vi "Quaternion_Equals.vi"(9 "Other Quaternion":T1={"R"=1.0, "V"=[0.0, 0.0, 0.0]}, 11 "Quaternion":T1={"R"=1.0, "V"=[0.0, 0.0, 0.0]}) -> (1 "Equal2":bool, 3 "Equal":bool)   [LabVIEW 2019, in "Trajectory_Library.lvlib"]
doc: "Convenience constructors that takes in x and y values directly instead of having to construct a Translation2d.\n\nParameters:\n - X- The x component of the translational component of the pose.\n - Y - The y component of the translational component of the pose.\n - Rotation (Heading) - The rotational component of the pose.\n\nReturns:\n - OUT POSE - Output POSE"
uses:
  Trajectory_Library.lvlib
  QUATERNION.ctl
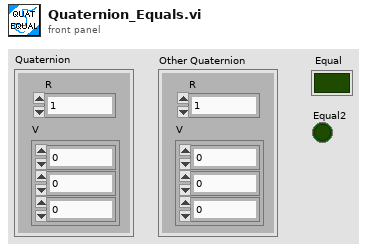
[diagram p1: front panel]
types:
  T1 = typedef "Trajectory_Library.lvlib/QUATERNION.ctl" = cluster{"R":dbl, "V":dbl[]}
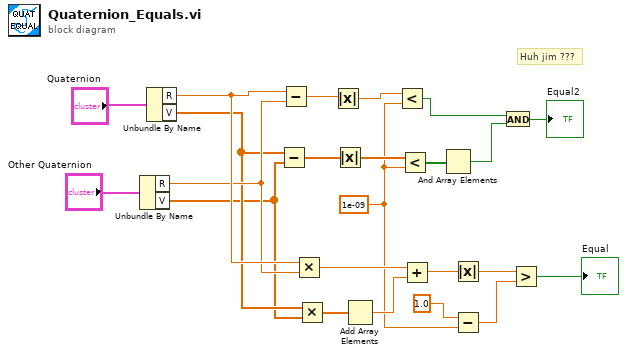
[diagram p0: block diagram]
diagram:
  w4 = 1e-09 ("y")
  # "Huh jim ???"
  n1 = Unbundle By Name("Other Quaternion") -> ("R"=w13:dbl, "V"=w11:dbl[])
  n2 = Unbundle By Name("Quaternion") -> ("R"=w14:dbl, "V"=w12:dbl[])
  n3 = Subtract(x=w12, y=w11) -> (x-y=w20:dbl[])
  n4 = Subtract(x=w14, y=w13) -> (x-y=w21:dbl)
  n5 = Multiply(x=w14, y=w13) -> (x*y=w9:dbl)
  n6 = Multiply(x=w12, y=w11) -> (x*y=w10:dbl[])
  n7 = Absolute Value(x=w21) -> (abs(x)=w19:dbl)
  n8 = Absolute Value(x=w20) -> (abs(x)=w18:dbl[])
  n9 = Add Array Elements(numeric array=w10) -> (sum=w8:dbl)
  n10 = Less?(x=w19, y=w4) -> (x < y?=w17:bool)
  n11 = Less?(x=w18, y=w4) -> (x < y?=w16:bool[])
  n12 = Add(x=w9, y=w8) -> (x+y=w7:dbl)
  n13 = And Array Elements(Boolean array=w16) -> (logical AND=w15:bool)
  n14 = Absolute Value(x=w7) -> (abs(x)=w6:dbl)
  n15 = Subtract(x=1.0, y=w4) -> (x-y=w3:dbl)
  n16 = And(x=w17, y=w15) -> (x .and. y?=→"Equal2":bool)
  n17 = Greater?(x=w6, y=w3) -> (0:→"Equal":bool)
